vi "Main IP V1.vi"() -> ()   [LabVIEW 2015]
uses:
  <vilib>/Utility/file.llb/Read Delimited Spreadsheet (string).vi
  Stream/LP Globals.vi
  <vilib>/Utility/file.llb/Write Delimited Spreadsheet (string).vi
panel:
  out "Grade":u32
  out "Image Dst Out":T1(plugin-control)
  in  "ExportTable":bool
  in  "Previous":bool
  in  "Base Path":path
  out "Picture Index":u16
  in  "Next":bool
  out "PicListFileNmae":path caption="Picture List File Nmae"
  in  "OpenPicList":bool
  in  "Pictures List":string[][](array[string])
  out "Closed":bool
  out "output cluster":T2
  out "Threshold Range Out":cluster{"Lower value":sgl, "Upper value":sgl}={"Lower value"=128.0, "Upper value"=255.0} {"Upper value" format="%.2f"; "Lower value" format="%.2f"}
  out "error out":errorcluster
  out "MaxY":u32
  out "MaxX":u32
  out "MaxB":u32
  out "MaxA":u32
  out "HorCenter":u16
  out "VerCenter":u32
  out "Image Out":T1(plugin-control)
  in  "Image Path":path=path "D:/BelkinVideos/f25_spacer3_vlad_190fps_1/Basler acA800-200gc (22058364)_20170111_114016323_0001.tiff"
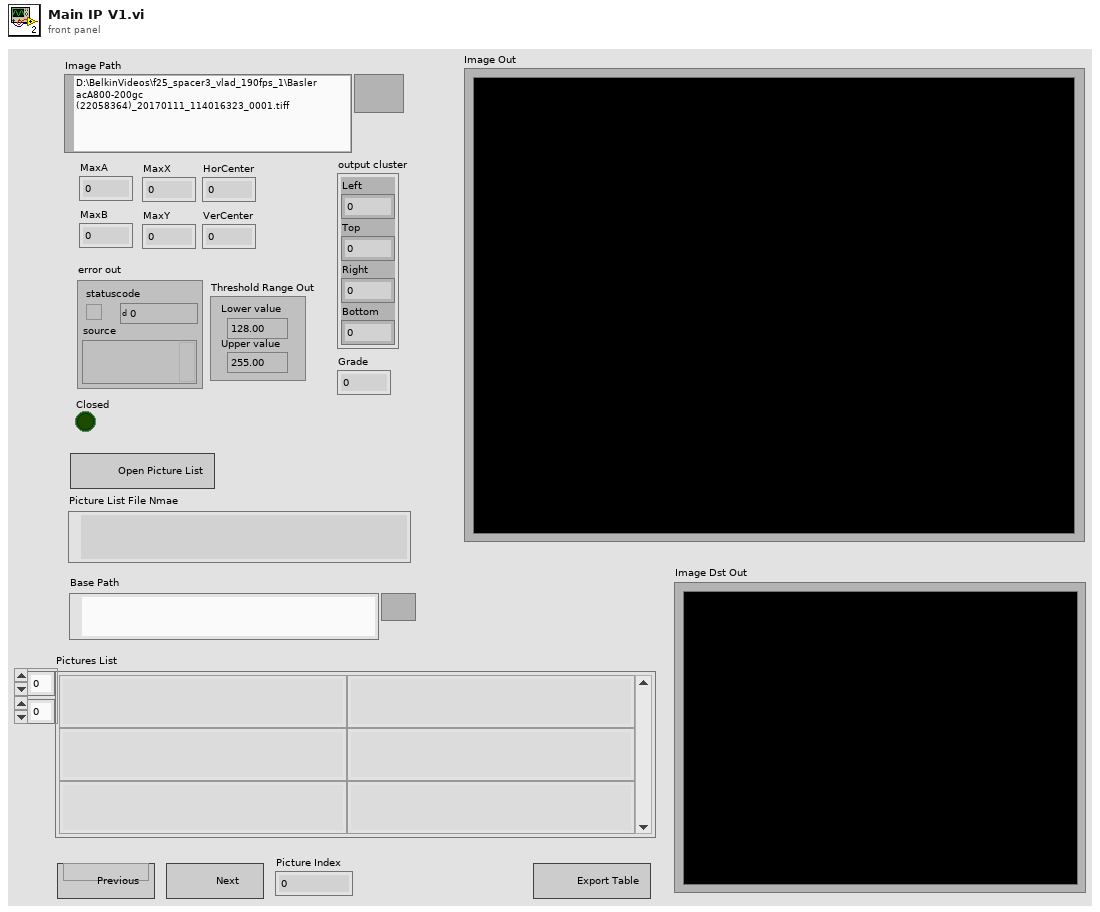
[diagram p1: front panel]
types:
  T1 = typedef "IMAQ Image.ctl" = refnum<image>
  T2 = cluster{"Left":i32, "Top":i32, "Right":i32, "Bottom":i32}
  T3 = typedef "Image Type" = u32
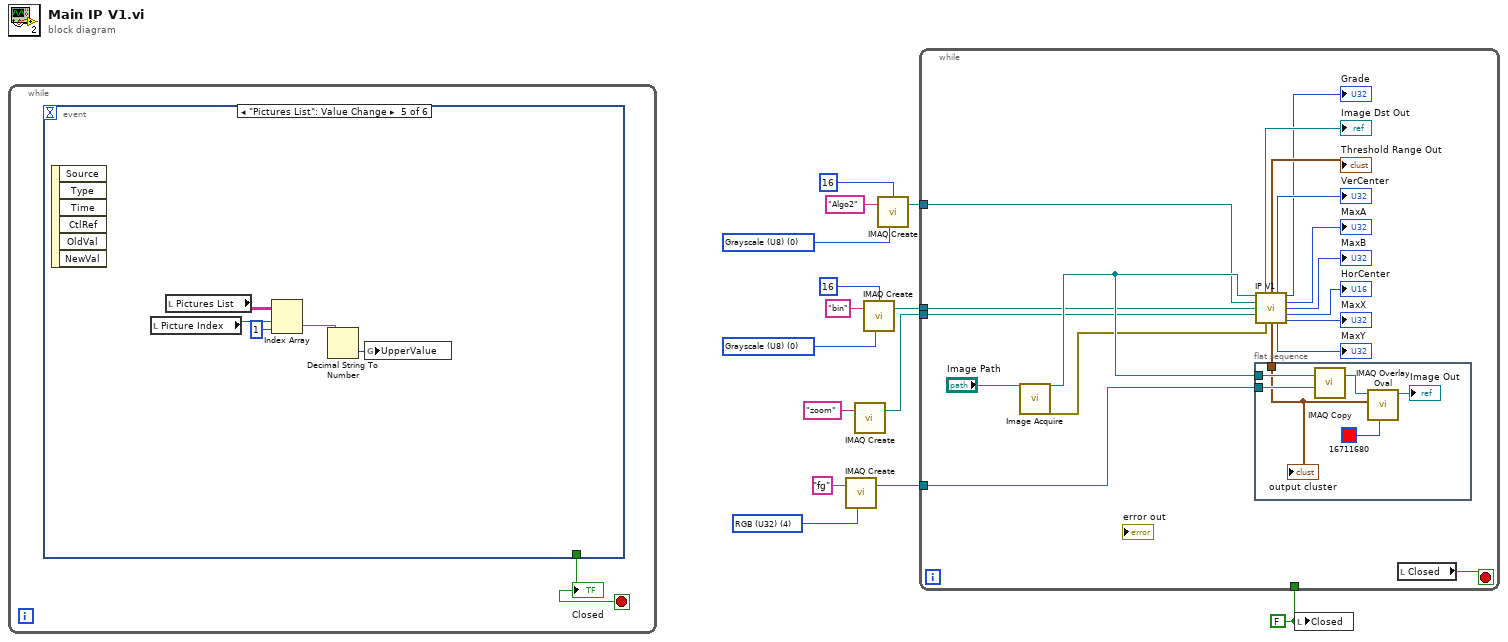
[diagram p0: block diagram]
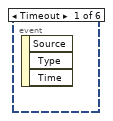
[diagram p2: hidden frame]
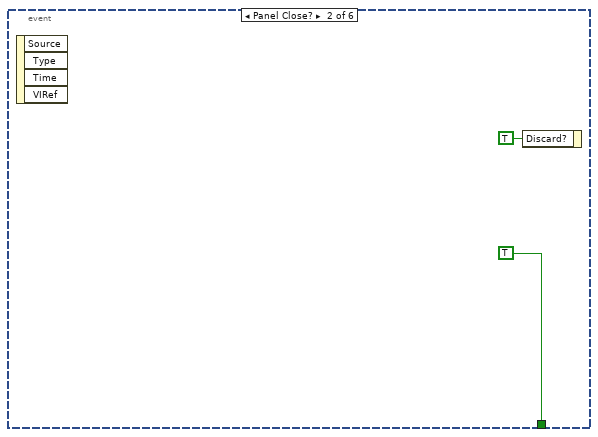
[diagram p3: hidden frame]
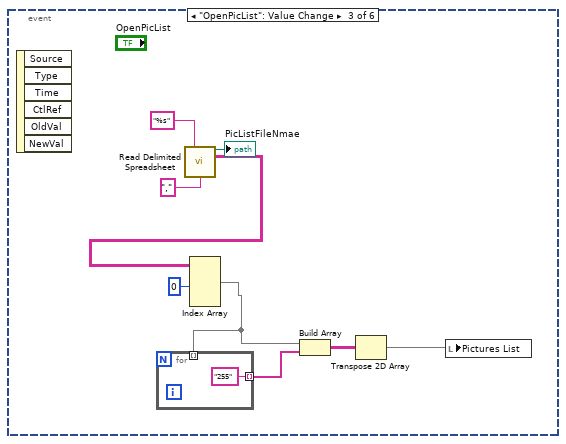
[diagram p4: hidden frame]
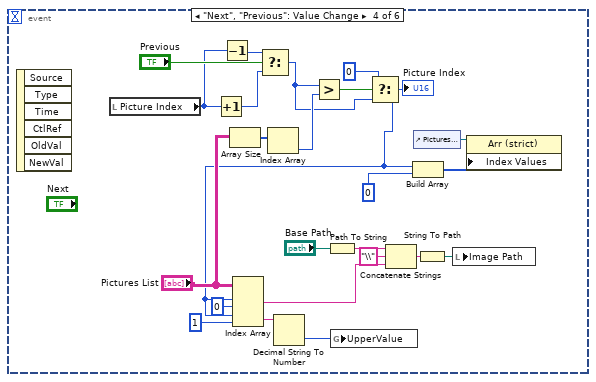
[diagram p5: hidden frame]
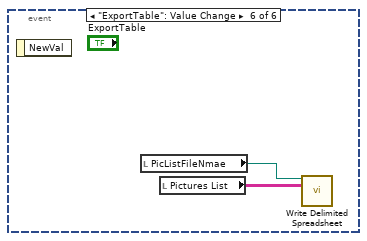
[diagram p6: hidden frame]
diagram:
  w1 = FALSE ("Closed")
  w8 = T3 0 items=["Grayscale (U8)", "Grayscale (I16)", "Grayscale (SGL)", "Complex (CSG)", "RGB (U32)", "HSL (U32)", "RGB (U64)", "Grayscale (U16)"] ("Image Type")
  w11 = T3 0 items=["Grayscale (U8)", "Grayscale (I16)", "Grayscale (SGL)", "Complex (CSG)", "RGB (U32)", "HSL (U32)", "RGB (U64)", "Grayscale (U16)"] ("Image Type")
  w13 = T3 4 items=["Grayscale (U8)", "Grayscale (I16)", "Grayscale (SGL)", "Complex (CSG)", "RGB (U32)", "HSL (U32)", "RGB (U64)", "Grayscale (U16)"] ("Image Type")
  n1 = while {
    stop <- w15 stop-if-true
    n2 = event shown="[4] \"Pictures List\": Value Change" {
      selector: _ -> [_ _ _ _ _ _]
      dyn-events: _ -> [_ _ _ _ _ _]
      timeout: _ -> [_ _ _ _ _ _]
      tunnel: [_ TRUE _ _ _ _] -> w15
      event Timeout {
        n3 = event-data() -> ()  [unwired: 1 in, 3 out]
      }
      event Panel Close? {
        n4 = event-data() -> ()  [unwired: 1 in, 4 out]
        n5 = event-data("Discard?"=TRUE) -> ()  [unwired: 1 in, 1 out]
      }
      event "OpenPicList": Value Change {
        n6 = event-data() -> ()  [unwired: 1 in, 6 out]
        n7 = call-poly <vilib>:"Read Delimited Spreadsheet.vi"("format (%s)"="%s", "delimiter (\\t)"="," ("delimiter (\\t)")) -> ("new file path (Not A Path if cancelled)"=→"PicListFileNmae":path, "all rows"=w20:string[][])  [unwired: 8 in, 4 out]
        n8 = Index Array(array=w20, index (col) #1=0 ("disabled index (col)")) -> (element #1=w22:string[])  [unwired: 3 in, 1 out]
        n9 = for {
          tunnel: w22 -> [_] mode=indexing
          tunnel: ["255"] -> w21 mode=indexing
        }
        n10 = Build Array(w22, w21) -> (w19:string[][])
        n11 = Transpose 2D Array(2D array=w19) -> (transposed array=w18:string[][])
        n12 = local write "Pictures List"(w18) -> ()
      }
      event "Next", "Previous": Value Change {
        n13 = event-data() -> ()  [unwired: 1 in, 6 out]
        n14 = local read "Picture Index"() -> (w29:u16)
        n15 = Increment(x=w29) -> (x+1=w36:u16)
        n16 = Decrement(x=w29) -> (x-1=w35:u16)
        n17 = Array Size(array="Pictures List") -> (size(s)=w40:i32[])
        n18 = Select(t=w35, s="Previous", f=w36) -> (s? t:f=w33:u16)
        n19 = Index Array(array=w40) -> (element=w39:i32)  [unwired: 1 in]
        n20 = Greater?(x=w33, y=w39) -> (0:w38:bool)
        n21 = Path To String(path="Base Path") -> (string=w43:string)
        n22 = Select(t=u16 0, s=w38, f=w33) -> (s? t:f=w28:u16)
        "Picture Index" <- w28
        n23 = Index Array(array="Pictures List", index (row) #1=w28, index (col) #1=0 ("disabled index (col)"), index (row) #2=w28, index (col) #2=1 ("disabled index (col)")) -> (element #1=w45:string, element #2=w49:string)
        n24 = Decimal String To Number(string=w49) -> (number=w48:i32)  [unwired: 2 in, 1 out]
        n25 = global write "LP Globals.vi" "UpperValue"(w48) -> ()
        n26 = Concatenate Strings(w43, "\\" ("string"), w45) -> (w44:string)
        n27 = Build Array(w28, u32 0) -> (w30:u32[])
        n28 = control-ref of="Pictures List"() -> (w32:refnum<vi>)
        n29 = String To Path(string=w44) -> (path=w47:path)
        n30 = local write "Image Path"(w47) -> ()
        n31 = property class="Arr (strict)"(reference=w32, "Index Values"=w30) -> ()  [unwired: 1 in, 2 out]
      }
      event "Pictures List": Value Change {
        n32 = event-data() -> ()  [unwired: 1 in, 6 out]
        n33 = local read "Picture Index"() -> (w53:u16)
        n34 = local read "Pictures List"() -> (w52:string[][])
        n35 = Index Array(array=w52, index (row)=w53, index (col)=1 ("disabled index (col)")) -> (element=w55:string)
        n36 = Decimal String To Number(string=w55) -> (number=w56:i32)  [unwired: 2 in, 1 out]
        n37 = global write "LP Globals.vi" "UpperValue"(w56) -> ()
      }
      event "ExportTable": Value Change {
        n38 = event-data() -> ()  [unwired: 1 in, 1 out]
        n39 = local read "PicListFileNmae"() -> (w57:path)
        n40 = local read "Pictures List"() -> (w58:string[][])
        n41 = call-poly <vilib>:"Write Delimited Spreadsheet.vi"("file path (dialog if empty)"=w57, "2D data"=w58) -> ()  [unwired: 12 in, 2 out]
      }
    }
    "Closed" <- w15
  }
  n42 = call "IMAQ Create"("Image Name"="fg", "Image Type"=w13) -> ("New Image"=w12:T1)  [unwired: 3 in, 1 out]
  n43 = call "IMAQ Create"("Image Name"="zoom") -> ("New Image"=w2:T1)  [unwired: 4 in, 1 out]
  n44 = call "IMAQ Create"("Border Size"=16, "Image Name"="bin", "Image Type"=w8) -> ("New Image"=w5:T1)  [unwired: 2 in, 1 out]
  n45 = call "IMAQ Create"("Border Size"=16, "Image Name"="Algo2", "Image Type"=w11) -> ("New Image"=w4:T1)  [unwired: 2 in, 1 out]
  n46 = while {
    tunnel: w12 -> [w71]
    tunnel: w5 -> [w68]
    tunnel: w4 -> [w67]
    tunnel: w2 -> [w63]
    tunnel: w1 -> [_]
    stop <- w62 stop-if-true
    n47 = call "Image Acquire.vi"("Image Path"="Image Path") -> ("Image Out"=w70:T1, "error out"=w61:errorcluster)  [unwired: 25 in]
    n48 = flat-sequence {
      tunnel: w71 -> [w80]
      tunnel: w70 -> [w79]
      tunnel: w69 -> [w77]
      frame #0 {
        n49 = call "IMAQ Copy"("Image Dst"=w80, "Image Src"=w79) -> ("Image Dst Out"=w78:T1)  [unwired: 1 in, 4 out]
        n50 = call "IMAQ Overlay Oval"("Color"=u32 16711680, "Bounding Rectangle"=w77, "Image"=w78) -> ("Image Out"=→"Image Out":T1)  [unwired: 7 in, 1 out]
        "output cluster" <- w77
      }
    }
    n51 = call "IP V1.vi"("Image In"=w70, "Image Dst"=w67, "BinImage"=w68, "Zoom Image"=w63, "error in"=w61) -> ("Image Dst Out"=→"Image Dst Out":T1, "Threshold Range Out"=→"Threshold Range Out":cluster{"Lower value":sgl, "Upper value":sgl}, "VerCenter"=→"VerCenter":u32, "MaxGrade"=→"Grade":u32, "MaxA"=→"MaxA":u32, "MaxB"=→"MaxB":u32, "HorCenter"=→"HorCenter":u16, "output cluster"=w69:T2, "MaxY"=→"MaxY":u32, "MaxX"=→"MaxX":u32)  [unwired: 1 out]
    n52 = local read "Closed"() -> (w62:bool)
  }
  n53 = local write "Closed"(w1) -> ()
